vi "trueFrameRate.set.vi"(8 "error in (no error)":errorcluster, 10 "trueFrameRate":dbl, 11 "trueFrameRate in":refnum<class "trueFrameRate.lvclass">) -> (0 "error out":errorcluster, 3 "trueFrameRate out":refnum<class "trueFrameRate.lvclass">)   [LabVIEW 2020, in "nominal types.lvlib" / "timestampManifest.lvlib" / "trueFrameRate.lvclass"]
uses:
  trueFrameRate.lvclass
  trueFrameRate.lvclass/trueFrameRate.ctl
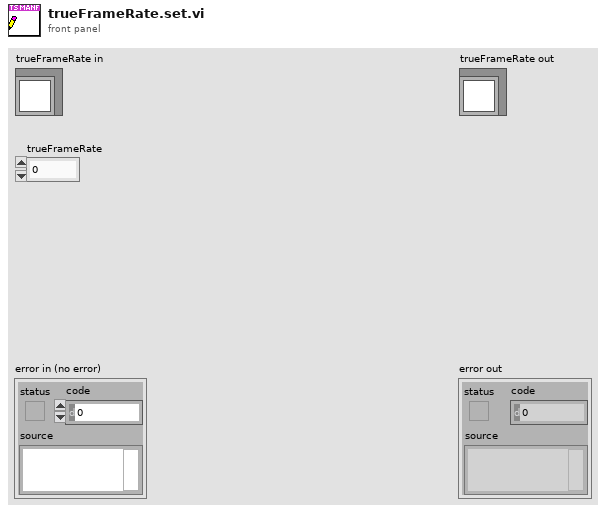
[diagram p1: front panel]
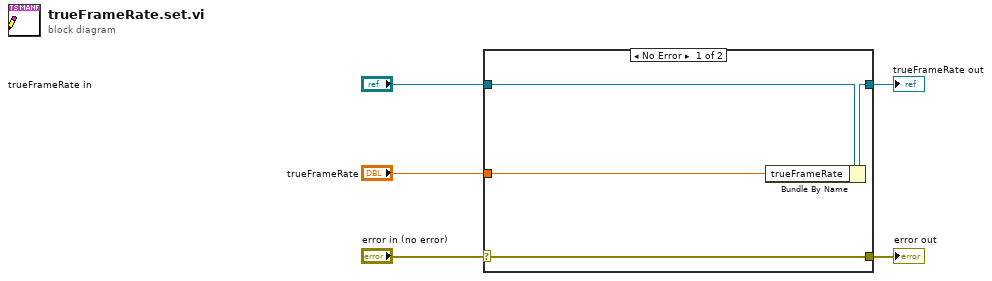
[diagram p0: block diagram]
diagram:
  n1 = case shown="No Error" "error in (no error)" {
    selector: "error in (no error)" -> [w9 w10]
    tunnel: [w9 w10] -> w4
    tunnel: [w7 w11] -> w2
    tunnel: "trueFrameRate in" -> [w8 w11]
    tunnel: "trueFrameRate" -> [w6 _]
    frame No Error {
      n2 = Bundle By Name(cluster=w8, "trueFrameRate"=w6) -> (w7:refnum<class "trueFrameRate.lvclass">)
    }
    frame Error {
    }
  }
  "error out" <- w4
  "trueFrameRate out" <- w2
